vi "GetZippedBookName.vi"(1 "Unzipped files":path[](array[path]), 2 "path":path) -> (0 "String":string)   [LabVIEW 2012]
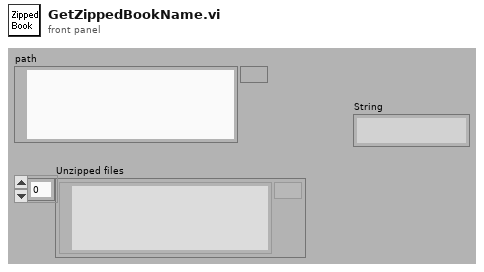
[diagram p1: front panel]
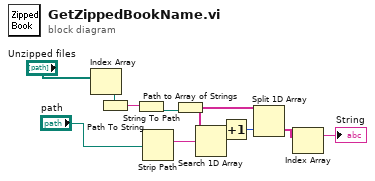
[diagram p0: block diagram]
diagram:
  n1 = Index Array(array="Unzipped files") -> (element=w10:path)  [unwired: 1 in]
  n2 = Path To String(path=w10) -> (string=w8:string)
  n3 = String To Path(string=w8) -> (path=w11:path)
  n4 = Strip Path(path="path") -> (name=w6:string)  [unwired: 1 out]
  n5 = Path to Array of Strings(0:w11) -> (2:w5:string[])  [unwired: 1 out]
  n6 = Search 1D Array(1D array=w5, element=w6) -> (index of element=w4:i32)  [unwired: 1 out]
  n7 = Increment(x=w4) -> (x+1=w1:i32)
  n8 = Split 1D Array(array=w5, index=w1) -> (second subarray=w3:string[])  [unwired: 1 out]
  n9 = Index Array(array=w3) -> (element=→"String":string)  [unwired: 1 in]
